vi "roboRIO v1.0 Open I2C.vi"(7 "Allow multiple opens?":bool, 8 "error in (no error)":errorcluster, 10 "Channel Name":string, 11 "Resource name":T1 caption="RIO Device") -> (0 "error out":errorcluster, 2 "I2C Channel":T2, 3 "myRIO Ref Out":T3)   [LabVIEW 2021]
uses:
  <vilib>/myRIO/Common/Instrument Driver Framework/Utilities/typedefs/myRIO v1.0 Reference.ctl
  <vilib>/myRIO/Common/Instrument Driver Framework/Utilities/typedefs/Generic FPGA Reference.ctl
  <vilib>/myRIO/Common/Instrument Driver Framework/myRIO v1.0/I2C/typedefs/I2C Channels Enum.ctl
  <vilib>/userDefined/High Color/nirio_resource_hc.ctl
  <vilib>/myRIO/Common/Instrument Driver Framework/roboRIO v1.0/I2C/typedefs/roboRIO v1.0 I2C Channels Enum.ctl
  <vilib>/myRIO/Common/Instrument Driver Framework/roboRIO v1.0/Resource Manager/vis/roboRIO v1.0 Reserve Channel List.vi
  <vilib>/myRIO/Common/Instrument Driver Framework/roboRIO v1.0/I2C/vis/roboRIO v1.0 Build MUX Configuration I2C.vi
  <vilib>/myRIO/Common/Instrument Driver Framework/roboRIO v1.0/Resource Manager/vis/roboRIO v1.0 Reserve Channel.vi
  <vilib>/myRIO/Common/Instrument Driver Framework/roboRIO v1.0/Resource Manager/vis/roboRIO v1.0 Unreserve Channel.vi
  <vilib>/myRIO/Common/Instrument Driver Framework/roboRIO v1.0/Resource Manager/vis/roboRIO v1.0 Create Configuration List.vi
  <vilib>/myRIO/Common/Instrument Driver Framework/roboRIO v1.0/Resource Manager/vis/roboRIO v1.0 Build Mutex Name.vi
  <vilib>/Utility/VariantDataType/GetNumericInfo.vi
  <vilib>/Utility/error.llb/Error Cluster From Error Code.vi
  <vilib>/myRIO/Common/Instrument Driver Framework/Utilities/vis/IO Manager.vi
  <vilib>/myRIO/Common/Instrument Driver Framework/Utilities/vis/Configuration Manager.vi
  <vilib>/myRIO/Common/Instrument Driver Framework/roboRIO v1.0/Resource Manager/vis/roboRIO v1.0 Configure IO.vi
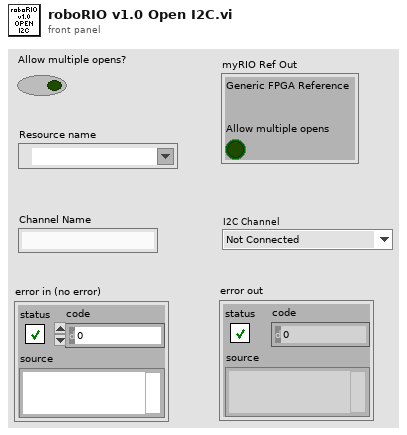
[diagram p1: front panel]
types:
  T1 = typedef "nirio_resource_hc.ctl" = tag
  T2 = typedef "I2C Channels Enum.ctl" = enum16{"Not Connected", "A/I2C", "B/I2C", "I2C/I2C"}
  T3 = typedef "myRIO v1.0 Reference.ctl" = cluster{"Generic FPGA Reference":T4, "Allow multiple opens":bool}
  T4 = typedef "Generic FPGA Reference.ctl" = refnum<k20>
  T5 = typedef "roboRIO v1.0 I2C Channels Enum.ctl" = enum16{"Not Connected", "B/I2C", "I2C/I2C"}
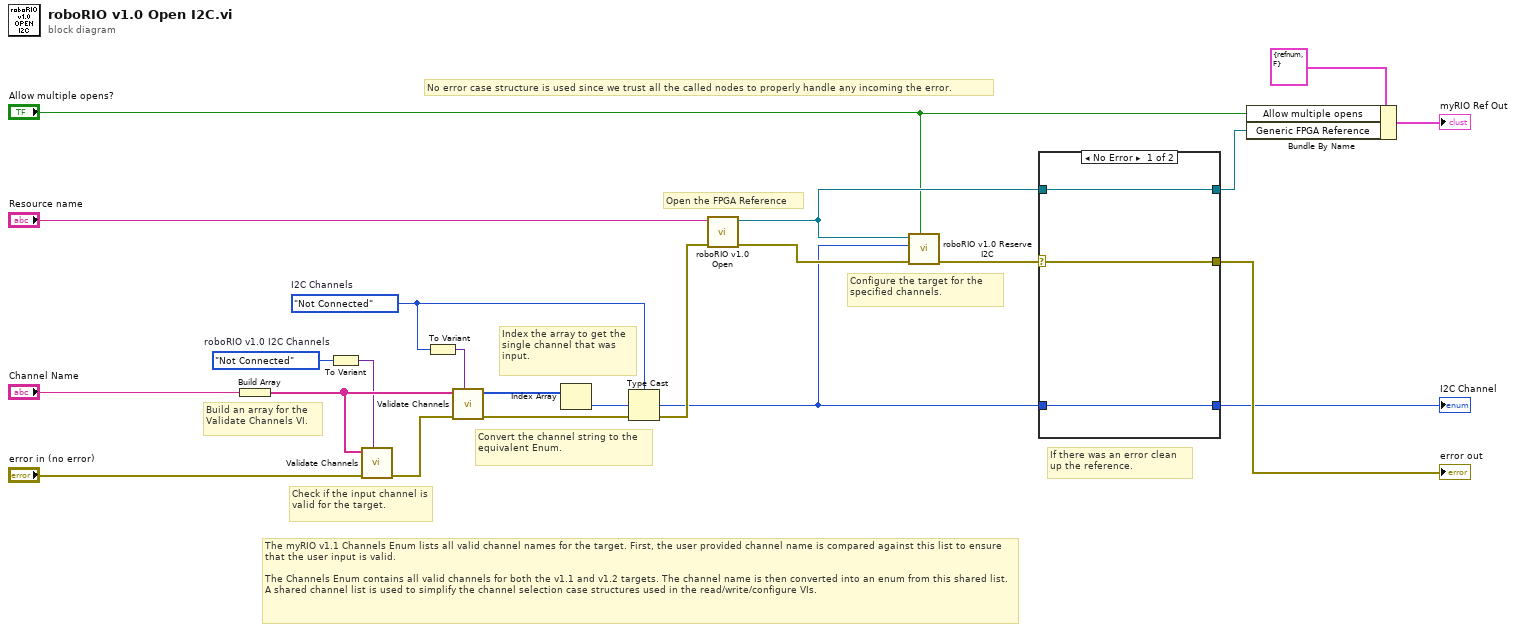
[diagram p0: block diagram]
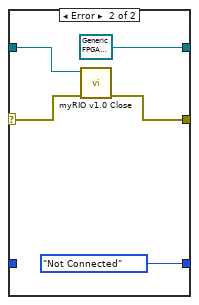
[diagram p2: hidden frame]
diagram:
  w2 = roboRIO_v1.0_I2C_Channels_Enum."Not Connected"  # roboRIO v1.0 I2C Channels
  w1 = I2C_Channels_Enum."Not Connected"  # I2C Channels
  # "The myRIO v1.1 Channels Enum lists all valid channel names for the target. First, the user provided channel name is compared against this list to ensure that the user input is valid.\n\nThe Channels Enum contains all valid channels for both the v1.1 and v1.2 targets. The channel name is then converted into an enum from this shared list. A shared channel list is used to simplify the channel selection case structures used in the read/write/configure VIs."
  # "Index the array to get the single channel that was input."
  # "Build an array for the Validate Channels VI."
  # "If there was an error clean up the reference."
  # "Configure the target for the specified channels."
  # "Open the FPGA Reference"
  # "No error case structure is used since we trust all the called nodes to properly handle any incoming the error."
  # "Convert the channel string to the equivalent Enum."
  # "Check if the input channel is valid for the target."
  n1 = Build Array("Channel Name") -> (w13:string[])
  n2 = To Variant(anything=w2) -> (Variant=w3:variant)
  n3 = call <vilib>:"Validate Channels.vi"("Channels Enum Variant"=w3, "error in (no error)"="error in (no error)", "Channel Names"=w13) -> ("error out"=w21:errorcluster)  [unwired: 7 in, 1 out]
  n4 = To Variant(anything=w1) -> (Variant=w4:variant)
  n5 = call <vilib>:"Validate Channels.vi"("Channels Enum Variant"=w4, "error in (no error)"=w21, "Channel Names"=w13) -> ("error out"=w18:errorcluster, "Index Array"=w12:u16[])  [unwired: 7 in]
  n6 = Index Array(array=w12) -> (element=w11:u16)  [unwired: 1 in]
  n7 = Type Cast(type=w1, x=w11) -> (*(type *) &x=w10:T2)
  n8 = call <vilib>:"roboRIO v1.0 Open.vi"("error in (no error)"=w18, "Resource name"="Resource name") -> ("error out"=w17:errorcluster, "myRIO FPGA Ref Out"=w15:T4)  [unwired: 8 in]
  n9 = call <vilib>:"roboRIO v1.0 Reserve I2C.vi"("Allow multiple opens?"="Allow multiple opens?", "error in (no error)"=w17, "I2C Channel"=w10, "myRIO FPGA Ref Out"=w15) -> ("error out"=w16:errorcluster)  [unwired: 7 in]
  n10 = case shown="No Error" w16 {
    selector: w16 -> [w24 w30]
    tunnel: w15 -> [w25 w28]
    tunnel: [w25 T4 refnum ("myRIO FPGA Ref Out")] -> w6
    tunnel: [w24 w29] -> w19
    tunnel: w10 -> [w23 _]
    tunnel: [w23 I2C_Channels_Enum."Not Connected"] -> w9
    frame No Error {
    }
    frame Error {
      n11 = call <vilib>:"myRIO v1.0 Close.vi"("error in (no error)"=w30, "myRIO FPGA Ref In"=w28) -> ("error out"=w29:errorcluster)  [unwired: 9 in]
    }
  }
  "I2C Channel" <- w9
  "error out" <- w19
  n12 = Bundle By Name(cluster=T3 {"Generic FPGA Reference"=refnum, "Allow multiple opens"=FALSE} ("myRIO v1.0 Reference"), "Allow multiple opens"="Allow multiple opens?", "Generic FPGA Reference"=w6) -> (→"myRIO Ref Out":T3)
